vi "Exercise1.2-Selector.vi"() -> ()   [LabVIEW 2013]
panel:
  out "Output":dbl
  in  "Input":dbl
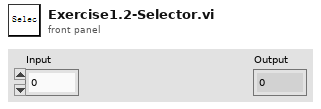
[diagram p1: front panel]
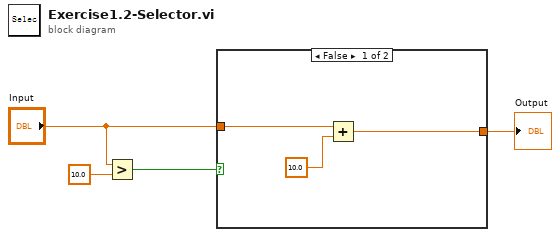
[diagram p0: block diagram]
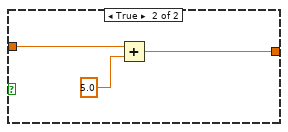
[diagram p2: hidden frame]
diagram:
  n1 = Greater?(x="Input", y=10.0) -> (0:w3:bool)
  n2 = case shown="False" w3 {
    tunnel: "Input" -> [w5 w10]
    tunnel: [w6 w8] -> w1
    frame False {
      n3 = Add(x=w5, y=10.0) -> (x+y=w6:dbl)
    }
    frame True {
      n4 = Add(x=w10, y=5.0) -> (x+y=w8:dbl)
    }
  }
  "Output" <- w1
